vi "Fetch git-describe tag version.vi"(8 "error in (no error)":errorcluster, 10 "git repo path":path=path "C:/", 11 "git.exe path":path=path "C:/Program Files/Git/cmd/git.exe") -> (0 "error out":errorcluster, 1 "Fetch error?":bool, 2 "Resolved version":T1, 3 "Version string":string)   [LabVIEW 2016]
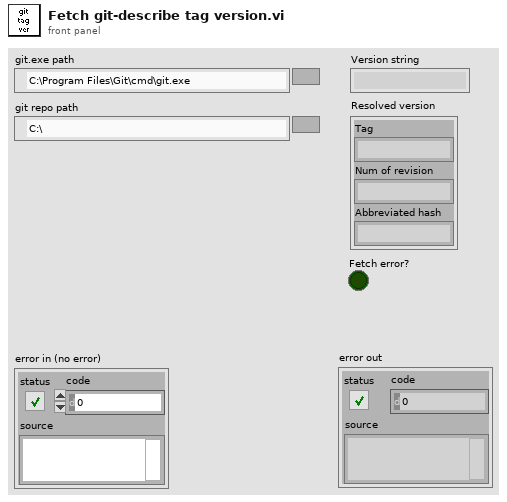
[diagram p1: front panel]
types:
  T1 = cluster{"Tag":string, "Num of revision":string, "Abbreviated hash":string}
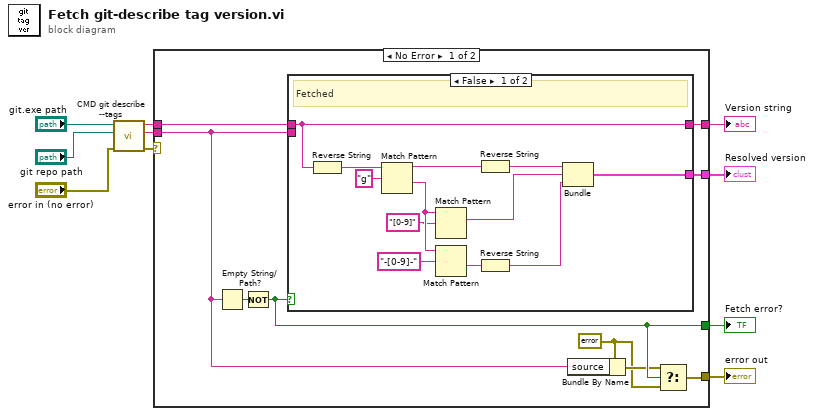
[diagram p0: block diagram]
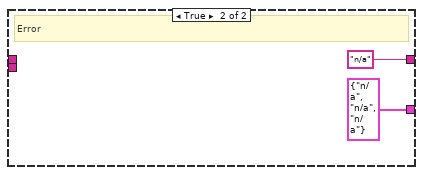
[diagram p2: hidden frame]
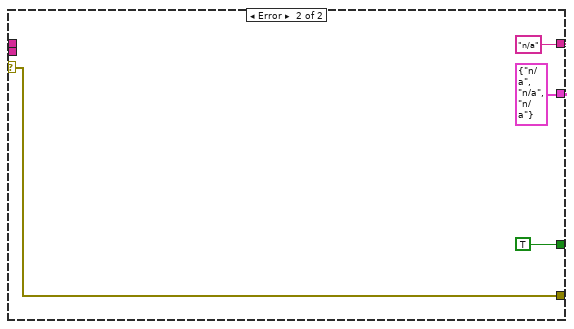
[diagram p3: hidden frame]
diagram:
  n1 = call "CMD git describe --tags.vi"("error in (no error)"="error in (no error)", "git repo path"="git repo path", "git.exe path"="git.exe path") -> ("error out"=w1:errorcluster, "standard error"=w2:string, "standard output"=w3:string)  [unwired: 5 in, 1 out]
  n2 = case shown="No Error" w1 {
    selector: w1 -> [_ w34]
    tunnel: [w19 TRUE] -> w10
    tunnel: [w18 w34] -> w9
    tunnel: [w17 "n/a" ("standard output")] -> w8
    tunnel: [w16 cluster{string, string, string} {"n/a", "n/a", "n/a"}] -> w7
    tunnel: w3 -> [w13 _]
    tunnel: w2 -> [w12 _]
    frame No Error {
      w11 = errorcluster {"status"=FALSE, "code"=0, "source"=""} ("error in (no error)")
      n3 = Empty String/Path?(string/path=w12) -> (empty?=w15:bool)
      n4 = Not(x=w15) -> (.not. x?=w19:bool)
      n5 = case shown="False" w19 {
        tunnel: w13 -> [w24 _]
        tunnel: [w24 "n/a" ("standard output")] -> w17
        tunnel: [w20 cluster{string, string, string} {"n/a", "n/a", "n/a"}] -> w16
        tunnel: w12 -> [_ _]
        frame False {
          # "Fetched"
          n6 = Reverse String(1:w24) -> (0:w25:string)
          n7 = Match Pattern(string=w25, regular expression="g") -> (before substring=w27:string, after substring=w30:string)  [unwired: 1 in, 2 out]
          n8 = Match Pattern(string=w30, regular expression="[0-9]") -> (match substring=w22:string)  [unwired: 1 in, 3 out]
          n9 = Match Pattern(string=w30, regular expression="-[0-9]-") -> (after substring=w31:string)  [unwired: 1 in, 3 out]
          n10 = Reverse String(1:w27) -> (0:w23:string)
          n11 = Reverse String(1:w31) -> (0:w21:string)
          n12 = Bundle(w23, w22, w21) -> (w20:cluster{string, string, string})  [unwired: 1 in]
        }
        frame True {
          # "Error"
        }
      }
      n13 = Bundle By Name(cluster=w11, "source"=w12) -> (w14:errorcluster)
      n14 = Select(t=w14, s=w19, f=w11) -> (s? t:f=w18:errorcluster)
    }
    frame Error {
    }
  }
  "Fetch error?" <- w10
  "error out" <- w9
  "Version string" <- w8
  "Resolved version" <- w7
